vi "Simulated Thermocouple RT Driver VI.vi"(6 "Device Clock":string, 9 "Device Inputs FIFO":refnum<k33>, 10 "Device Outputs FIFO":refnum<k33>, 11 "Device Reference":T1 format="%.0x") -> ()   [LabVIEW 2011, in "Simulated Thermocouple Custom Device.lvlib"]
uses:
  Simulated Thermocouple Custom Device.lvlib
  <vilib>/NI Veristand/Custom Device API/Custom Device Item Ref.ctl
  <vilib>/NI Veristand/Custom Device API/Custom Device Channel Type.ctl
  RT TC Update State.ctl
  <vilib>/Platform/TimedLoop/XDataNode/timing_clust.ctl
  <vilib>/Platform/TimedLoop/XDataNode/nitl_modes.ctl
  <vilib>/Platform/TimedLoop/XDataNode/wakeup.ctl
  <vilib>/NI Veristand/Custom Device API/Message Response (String).ctl
  <vilib>/NI Veristand/Custom Device API/Message Response (Byte Array).ctl
  <vilib>/DAQmx/write.llb/DAQmx Write (Analog 1D DBL NChan 1Samp).vi
  <vilib>/DAQmx/miscellaneous.llb/DAQmx Fill In Error Info.vi
  <vilib>/Platform/TimedLoop/XDataNode/XDataNode.xnode
  <vilib>/NI Veristand/Custom Device API/Custom Device API.lvlib
  <vilib>/NI Veristand/Custom Device Tools/Custom Device Utility Library/Custom Device Utility Library.lvlib
  <vilib>/Platform/TimedLoop/XDataNode/XDNodeRunTimeDep.lvlib
panel:
  in  "Initialization Status Notifier":refnum<notifier>
  in  "Status Notifier":refnum<notifier>
  # "Custom Device Template\nv1.0"
  # "Use this template as a starting point for creating a custom device code module. The input controls shown here are specially named controls that the system will use to provide the device loop with data. The controls are not required for the device loop to run. For instance, if the device doesn't produce any output data, then you don't need the Device Outputs FIFO control. If you do use these controls, however, they need to have these exact names to be functional."
  # "The optional status notifier element is used to notify the RT engine of the last state of the custom device, and to indicate the device has completed execution. If this control is not used, a default No Error value is returned to the system when the device finishes execution.\n\nNote: This error state is not checked until the system shuts down. Use an output status channel to send more immediate status values to the system."
  # "This optional input can be used to send the VeriStand Engine the final status of the custom device initalization process. If this control exists on the custom device front panel, the VeriStand Engine will wait for a status update before starting up. If the custom device reports an error, that will abort the execution of the current configuration in the VeriStand Engine.\n\nThis control can be deleted if the custom device does not need to send the initialization status update."
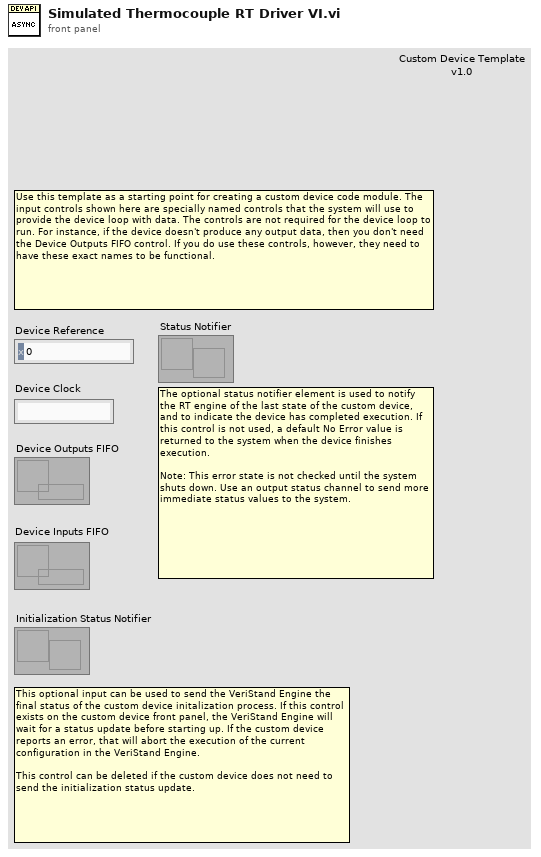
[diagram p1: front panel]
types:
  T1 = typedef "Custom Device API.lvlib/Custom Device Item Ref.ctl" = u64
  T2 = typedef "Custom Device API.lvlib/Custom Device Channel Type.ctl" = enum16{"Input", "Output"}
  T3 = typedef "Custom Device API.lvlib/Custom Device Timed Loop Priority.ctl" = enum32{"Low", "Medium", "High"}
  T4 = typedef "Custom Device API.lvlib/Custom Device Engine Event Ref.ctl" = refnum<event-registration>
  T5 = typedef "Simulated Thermocouple Custom Device.lvlib/RT Config Data.ctl" = cluster{"Current Task":refnum<k21>, "Voltage Task":refnum<k21>, "FIFO Sort Key":enum16{"SimTC", "Calibration", "VO", "CO"}[], "Cal Channel Indicies":i32[], "Current Initial Values":dbl[], "Voltage Initial Values":dbl[], "TC Channel Config":T6[], "TC Update Period":dbl, "Voltage Divider Ratio":dbl, "Samples To Collect":dbl, "Temperature Units":T8, "Cal Settling Time":dbl, "Cal Types":T7[]}
  T6 = typedef "Simulated Thermocouple Custom Device.lvlib/TC Channel Config Data.ctl" = cluster{"Thermocouple Type":T7, "Temperature Units":T8}
  T7 = typedef "Simulated Thermocouple Custom Device.lvlib/TC Selector.ctl" = u16
  T8 = typedef "Simulated Thermocouple Custom Device.lvlib/TC Unit Selector.ctl" = u16
  T9 = typedef "Simulated Thermocouple Custom Device.lvlib/RT TC Update State.ctl" = enum16{"Init", "Calibrate", "Update", "Idle"}
  T10 = typedef "XDNodeRunTimeDep.lvlib/timing_clust.ctl" = cluster{"Expected End [f-1]":u64, "Actual End [f-1]":u64, "Finished Late? [f-1]":bool, "Expected End [i-1]":u64, "Actual End [i-1]":u64, "Finished Late? [i-1]":bool, "Expected Start [i]":u64, "Actual Start [i]":u64, "Expected Start [f]":u64, "Actual Start [f]":u64, "Source Name":string, "Structure Name":string, "Period":i64, "Deadline":i64, "Offset":i64, "Start":i64, "Priority":i32, "Timeout":i32, "Mode":T11, "Wakeup Reason":T12, "Error":errorcluster, "Source Type":string, "Secondary Source Type":string, "Global End Time":u64, "Global Start Time":u64, "Frame Duration":u64, "Iteration Duration":u64, "Assigned CPU":i32, "I/O Scan Engine Mode":u32}
  T11 = typedef "XDNodeRunTimeDep.lvlib/nitl_modes.ctl" = enum32{"No Change", "Process missed periods, maintain original phase", "Discard missed periods, maintain original phase", "Process missed periods, ignore original phase", "Discard missed periods, ignore original phase"}
  T12 = typedef "XDNodeRunTimeDep.lvlib/wakeup.ctl" = enum32{"Normal", "Aborted", "Asynchronous wakeup", "Timing source error", "Timed loop error", "Timeout"}
  T13 = typedef "Custom Device API.lvlib/Message Response (String).ctl" = cluster{"Response":string, "Error":errorcluster}
  T14 = typedef "Custom Device API.lvlib/Message Response (Byte Array).ctl" = cluster{"Response":u8[], "Error":errorcluster}
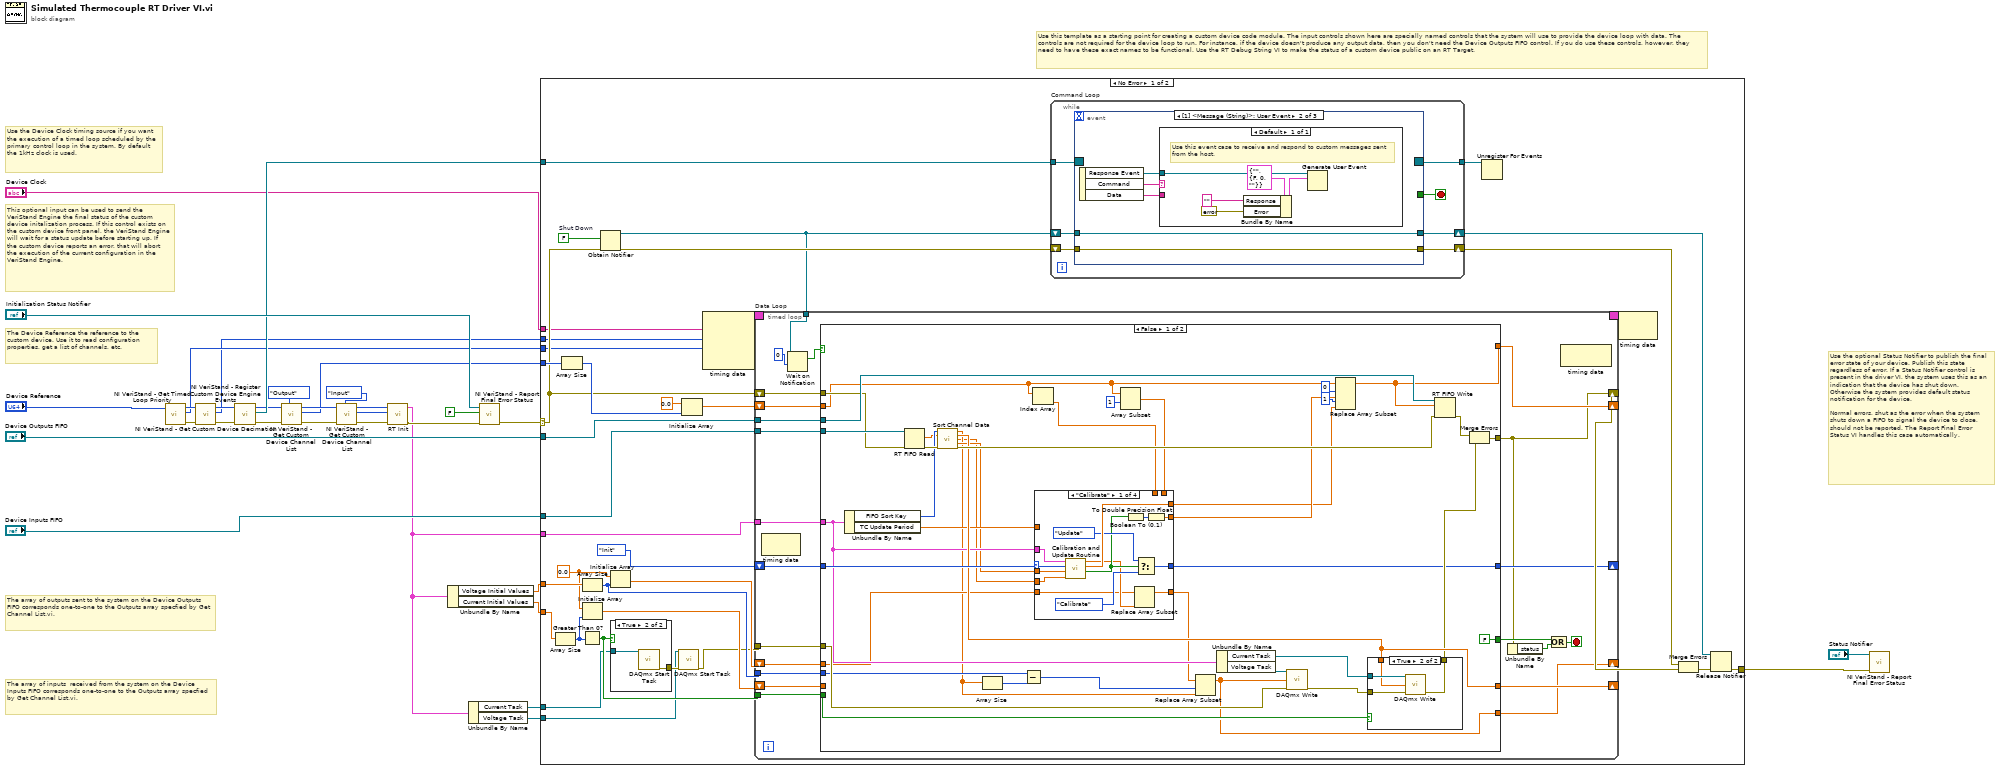
[diagram p0: block diagram]
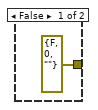
[diagram p2: hidden frame]
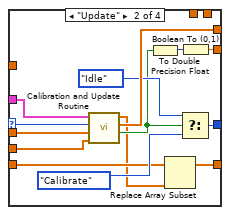
[diagram p4: hidden frame]
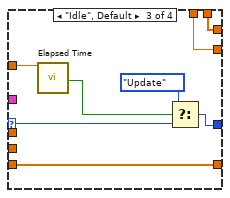
[diagram p5: hidden frame]
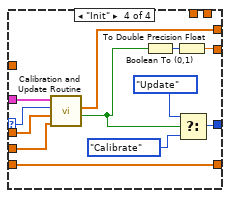
[diagram p6: hidden frame]
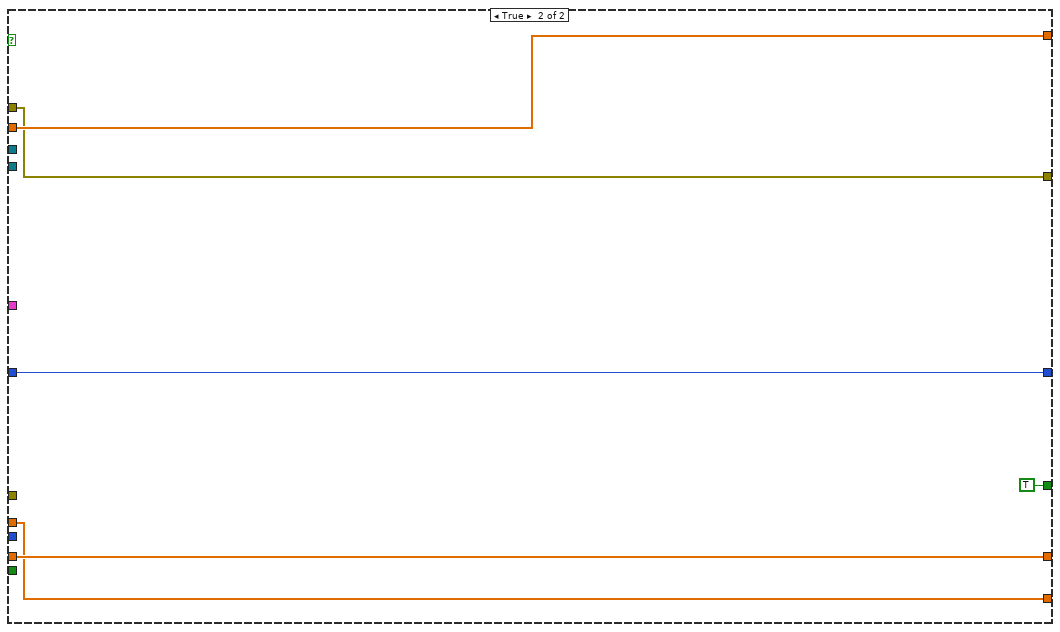
[diagram p7: hidden frame]
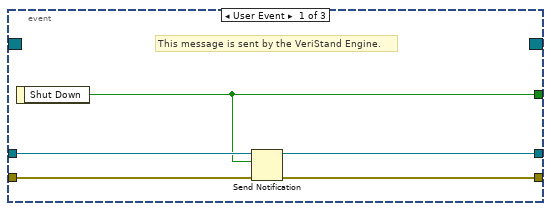
[diagram p8: hidden frame]
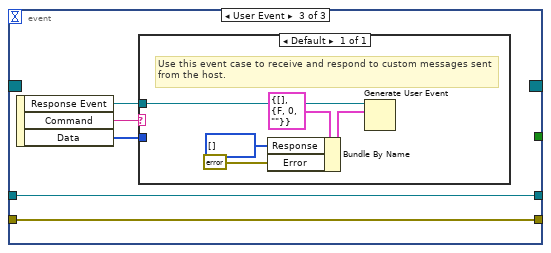
[diagram p9: hidden frame]
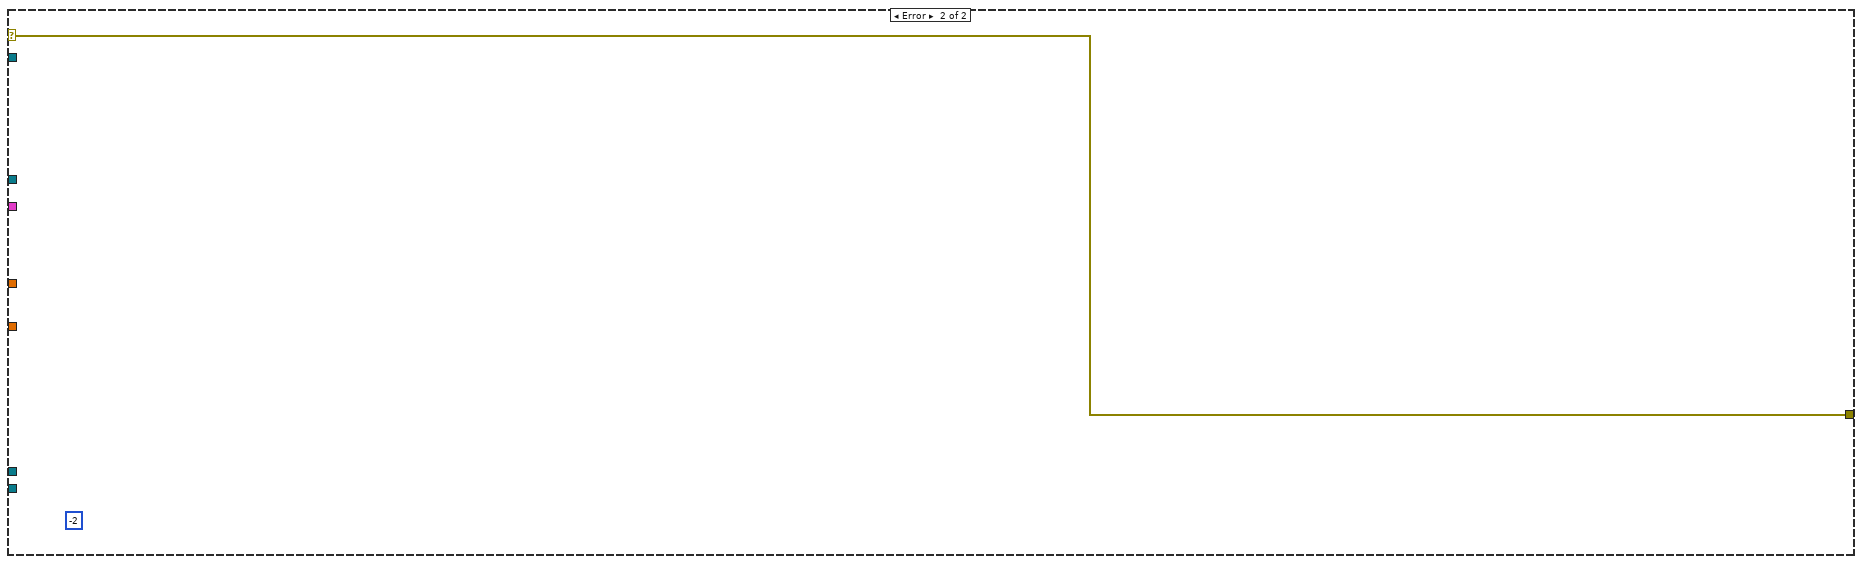
[diagram p10: hidden frame]
diagram:
  # "This optional input can be used to send the VeriStand Engine the final status of the custom device initalization process. If this control exists on the custom device front panel, the VeriStand Engine will wait for a status update before starting up. If the custom device reports an error, that will abort the execution of the current configuration in the VeriStand Engine."
  # "The array of inputs  received from the system on the Device Inputs FIFO corresponds one-to-one to the Outputs array specfied by Get Channel List.vi."
  # "Use the optional Status Notifier to publish the final error state of your device. Publish this state regardless of error. If a Status Notifier control is present in the driver VI, the system uses this as an indication that the device has shut down. Otherwise the system provides default status notification for the device.\n\nNormal errors, shut as the error when the system shuts down a FIFO to signal the device to close, should not be reported. The Report Final Error Status VI handles this case automatically."
  # "The array of outputs sent to the system on the Device Outputs FIFO corresponds one-to-one to the Outputs array specfied by Get Channel List.vi."
  # "The Device Reference the reference to the custom device. Use it to read configuration properties, get a list of channels, etc."
  # "Use the Device Clock timing source if you want the execution of a timed loop scheduled by the primary control loop in the system. By default the 1kHz clock is used."
  # "Use this template as a starting point for creating a custom device code module. The input controls shown here are specially named controls that the system will use to provide the device loop with data. The controls are not required for the device loop to run. For instance, if the device doesn't produce any output data, then you don't need the Device Outputs FIFO control. If you do use these controls, however, they need to have these exact names to be functional. Use the RT Debug String VI to make the status of a custom device public on an RT Target."
  n1 = call <vilib>:"NI VeriStand - Get Timed Loop Priority.vi"("Device Ref in"="Device Reference") -> ("error out"=w16:errorcluster, "Priority"=w4:T3, "Device Ref out"=w15:T1)  [unwired: 8 in]
  n2 = call <vilib>:"NI VeriStand - Get Custom Device Decimation.vi"("error in (no error)"=w16, "Device Ref in"=w15) -> ("error out"=w18:errorcluster, "Decimation"=w3:i32, "Device Ref out"=w17:T1)  [unwired: 7 in]
  n3 = call <vilib>:"NI VeriStand - Register Custom Device Engine Events.vi"("error in (no error)"=w18, "Device Ref in"=w17) -> ("error out"=w32:errorcluster, "Custom Device Engine Event Ref"=w23:T4, "Device Ref out"=w21:T1)  [unwired: 7 in]
  n4 = call <vilib>:"NI VeriStand - Get Custom Device Channel List.vi"("Channel Type"=Custom_Device_Channel_Type."Output", "error in (no error)"=w32, "Device Ref in"=w21) -> ("error out"=w26:errorcluster, "Specified Channel Ref List"=w19:T1[], "Device Ref out"=w27:T1)  [unwired: 6 out]
  n5 = call <vilib>:"NI VeriStand - Get Custom Device Channel List.vi"("Channel Type"=Custom_Device_Channel_Type."Input", "error in (no error)"=w26, "Device Ref in"=w27) -> ("error out"=w14:errorcluster, "Specified Channel Ref List"=w11:T1[], "Device Ref out"=w12:T1)  [unwired: 6 out]
  n6 = call "RT Init.vi"("error in"=w14, "Input Channels"=w11, "Custom Device Ref in"=w12) -> ("error out"=w13:errorcluster, "RT Configuration Data"=w7:T5)  [unwired: 7 in]
  n7 = Unbundle By Name(w7) -> ("Voltage Initial Values"=w9:dbl[], "Current Initial Values"=w8:dbl[])
  n8 = Unbundle By Name(w7) -> ("Current Task"=w6:refnum<k21>, "Voltage Task"=w5:refnum<k21>)
  n9 = call <vilib>:"NI VeriStand - Report Final Error Status.vi"("error in (no error)"=w13, "Filter FIFO Errors (T)"=FALSE, "Status Notifier"="Initialization Status Notifier") -> ("error out"=w20:errorcluster)  [unwired: 8 out]
  n10 = case shown="No Error" w20 {
    selector: w20 -> [w43 w232]
    tunnel: "Device Outputs FIFO" -> [w67 _]
    tunnel: "Device Inputs FIFO" -> [w66 _]
    tunnel: w19 -> [w62 _]
    tunnel: w23 -> [w61 _]
    tunnel: [w59 w232] -> w22
    tunnel: w7 -> [w41 _]
    tunnel: w9 -> [w50 _]
    tunnel: w8 -> [w49 _]
    tunnel: w6 -> [w37 _]
    tunnel: w5 -> [w36 _]
    tunnel: "Device Clock" -> [w35 _]
    tunnel: w4 -> [w34 _]
    tunnel: w3 -> [w33 _]
    frame No Error {
      w48 = 0.0 ("element")
      w60 = FALSE  # Shut Down
      n11 = Array Size(array=w49) -> (size(s)=w45:i32)
      n12 = Array Size(array=w62) -> (size(s)=w63:i32)
      n13 = Greater Than 0?(x=w45) -> (x > 0?=w38:bool)
      n14 = Array Size(array=w50) -> (size(s)=w44:i32)
      n15 = Initialize Array(w48, w45) -> (w46:dbl[])
      n16 = Obtain Notifier(notification data type=w60, error in (no error)=w43) -> (notifier out=w57:refnum<notifier>, error out=w68:errorcluster)  [unwired: 2 in, 1 out]
      n17 = Initialize Array(w48, w44) -> (w47:dbl[])
      n18 = case shown="True" w38 {
        tunnel: [errorcluster {"status"=FALSE, "code"=0, "source"=""} ("error out") w71] -> w39
        tunnel: w37 -> [_ w70]
        frame False {
        }
        frame True {
          n19 = call <vilib>:"DAQmx Start Task.vi"("task/channels in"=w70) -> ("error out"=w71:errorcluster)  [unwired: 13 in, 1 out]
        }
      }
      n20 = call <vilib>:"DAQmx Start Task.vi"("task/channels in"=w36, "error in"=w39) -> ("error out"=w40:errorcluster)  [unwired: 12 in, 1 out]
      n21 = Initialize Array(0.0 ("element"), w63) -> (w64:dbl[])
      n22 = node-c288(w35, w33, w34) -> (w53:T10)  [unwired: 1 in]
      n23 = timed-loop "Data Loop" {
        shift-right: [w92] -> _
        shift-left: w64 -> [w93]
        tunnel: w67 -> [w91]
        tunnel: w66 -> [w90]
        tunnel: w57 -> [w88]
        timing: w53 -> [_]
        timing-out: [_] -> w52
        tunnel: w41 -> [w85]
        shift-right: [w78] -> _
        shift-left: RT_TC_Update_State."Init" ("Enum") -> [w83]
        shift-right: [w79] -> _
        shift-left: w47 -> [w82]
        shift-right: [w80] -> _
        shift-left: w46 -> [w76]
        tunnel: w38 -> [w84]
        tunnel: w44 -> [w81]
        shift-right: [w75] -> w42
        shift-left: w43 -> [w77]
        tunnel: w40 -> [w73]
        stop <- w74 stop-if-true
        n24 = node-c288() -> ()  [unwired: 1 in, 1 out]
        n25 = Wait on Notification(notifier=w88, timeout in ms (-1)=0) -> (notification=w87:bool)  [unwired: 2 in, 3 out]
        n26 = case shown="False" w87 {
          tunnel: w93 -> [w110 w193]
          tunnel: [w114 w193] -> w92
          tunnel: w91 -> [w134 _]
          tunnel: w90 -> [w133 _]
          tunnel: [FALSE TRUE] -> w86
          tunnel: w85 -> [w117 _]
          tunnel: [w121 w191] -> w75
          tunnel: w84 -> [w128 _]
          tunnel: w83 -> [w126 w190]
          tunnel: w82 -> [w111 w188]
          tunnel: w81 -> [w100 _]
          tunnel: [w125 w189] -> w80
          tunnel: [w101 w188] -> w79
          tunnel: [w105 w190] -> w78
          tunnel: w77 -> [w122 w191]
          tunnel: w76 -> [_ w189]
          tunnel: w73 -> [w118 _]
          frame False {
            n27 = Unbundle By Name(w117) -> ("FIFO Sort Key"=w130:enum16{"SimTC", "Calibration", "VO", "CO"}[], "TC Update Period"=w123:dbl)
            n28 = RT FIFO Read(0:w133, 3:w122) -> (9:w113:dbl[], 11:w132:errorcluster)  [unwired: 1 in, 4 out]
            n29 = call "Sort Channel Data.vi"("Key"=w130, "Input Data"=w113, "error in (no error)"=w132) -> ("VO Channels"=w99:dbl[], "CO Channels"=w125:dbl[], "SimTC Channels"=w96:dbl[], "Calibration Channels"=w103:dbl[], "error out"=w129:errorcluster)  [unwired: 8 in]
            n30 = Array Size(array=w99) -> (size(s)=w98:i32)
            n31 = Subtract(x=w100, y=w98) -> (x-y=w97:i32)
            n32 = Index Array(array=w110) -> (element=w107:dbl)  [unwired: 1 in]
            n33 = Array Subset(array=w110, index=1) -> (w108:dbl[])  [unwired: 1 in]
            n34 = case shown="\"Calibrate\"" w126 {
              selector: w126 -> [w153 w166 w174 w186]
              tunnel: w111 -> [w140 w155 w168 w183]
              tunnel: [w142 w156 w168 w183] -> w102
              tunnel: w123 -> [_ _ w175 _]
              tunnel: [w147 w158 w171 w176] -> w105
              tunnel: w96 -> [w150 w164 _ w184]
              tunnel: w117 -> [w152 w167 _ w187]
              tunnel: w103 -> [w151 w165 _ w185]
              tunnel: [w149 w163 w169 w182] -> w104
              tunnel: [w143 w162 w170 w180] -> w106
              tunnel: w108 -> [_ _ w169 _]
              tunnel: w107 -> [_ _ w170 _]
              frame "Calibrate" {
                n35 = call "Calibration and Update Routine.vi"("simTC Channels"=w150, "Cal Channels"=w151, "TC Update State"=w153, "RT Configuration Data"=w152) -> ("Cal Valid?"=w145:bool, "Error"=w149:dbl[], "Voltages to Output"=w141:dbl[])  [unwired: 5 in]
                n36 = Boolean To (0,1)(Boolean=w145) -> (0, 1=w144:i16)
                n37 = Replace Array Subset(array=w140, new element=w141) -> (w142:dbl[])  [unwired: 1 in]
                n38 = Select(t=RT_TC_Update_State."Update" ("Enum"), s=w145, f=RT_TC_Update_State."Calibrate") -> (s? t:f=w147:T9)
                n39 = To Double Precision Float(number=w144) -> (double precision float=w143:dbl)
              }
              frame "Update" {
                n40 = call "Calibration and Update Routine.vi"("simTC Channels"=w164, "Cal Channels"=w165, "TC Update State"=w166, "RT Configuration Data"=w167) -> ("Cal Valid?"=w159:bool, "Error"=w163:dbl[], "Voltages to Output"=w154:dbl[])  [unwired: 5 in]
                n41 = Boolean To (0,1)(Boolean=w159) -> (0, 1=w161:i16)
                n42 = Replace Array Subset(array=w155, new element=w154) -> (w156:dbl[])  [unwired: 1 in]
                n43 = Select(t=RT_TC_Update_State."Idle" ("Enum"), s=w159, f=RT_TC_Update_State."Calibrate") -> (s? t:f=w158:T9)
                n44 = To Double Precision Float(number=w161) -> (double precision float=w162:dbl)
              }
              frame "Idle", Default {
                n45 = call "Elapsed Time"("Time Target (s)"=w175) -> ("Time has Elapsed"=w172:bool)  [unwired: 11 in, 7 out]
                n46 = Select(t=RT_TC_Update_State."Update", s=w172, f=w174) -> (s? t:f=w171:T9)
              }
              frame "Init" {
                n47 = call "Calibration and Update Routine.vi"("simTC Channels"=w184, "Cal Channels"=w185, "TC Update State"=w186, "RT Configuration Data"=w187) -> ("Cal Valid?"=w177:bool, "Error"=w182:dbl[])  [unwired: 5 in, 1 out]
                n48 = Boolean To (0,1)(Boolean=w177) -> (0, 1=w181:i16)
                n49 = To Double Precision Float(number=w181) -> (double precision float=w180:dbl)
                n50 = Select(t=RT_TC_Update_State."Update", s=w177, f=RT_TC_Update_State."Calibrate" ("Enum")) -> (s? t:f=w176:T9)
              }
            }
            n51 = Replace Array Subset(array=w102, new element=w99, index=w97) -> (w101:dbl[])
            n52 = Unbundle By Name(w117) -> ("Current Task"=w127:refnum<k21>, "Voltage Task"=w124:refnum<k21>)
            n53 = call-poly <vilib>:"DAQmx Write.vi"("task/channels in"=w124, "data"=w101, "error in"=w118) -> ("error out"=w112:errorcluster)  [unwired: 10 in, 2 out]
            n54 = Replace Array Subset(array=w110, new element #1=w106, index #1=0 ("index"), new element #2=w104, index #2=1 ("index")) -> (w114:dbl[])
            n55 = case shown="True" w128 {
              tunnel: w127 -> [_ w139]
              tunnel: w125 -> [_ w138]
              tunnel: w112 -> [w135 w137]
              tunnel: [w135 w136] -> w119
              frame False {
              }
              frame True {
                n56 = call-poly <vilib>:"DAQmx Write.vi"("task/channels in"=w139, "data"=w138, "error in"=w137) -> ("error out"=w136:errorcluster)  [unwired: 10 in, 2 out]
              }
            }
            n57 = RT FIFO Write(0:w134, 1:w114, 3:w129) -> (11:w120:errorcluster)  [unwired: 1 in, 4 out]
            n58 = Merge Errors(w120, w119) -> (w121:errorcluster)
          }
          frame True {
          }
        }
        n59 = Unbundle By Name(w75) -> ("status"=w72:bool)
        n60 = Compound Arithmetic op=OR(w86, w72) -> (w74:bool)
        n61 = node-c288() -> ()  [unwired: 1 in, 1 out]
      }
      n62 = while "Command Loop" {
        tunnel: w61 -> [w206]
        tunnel: [w205] -> w58
        shift-right: [w202] -> w56
        shift-left: w57 -> [w203]
        shift-right: [w200] -> w54
        shift-left: w68 -> [w201]
        stop <- w204 stop-if-true
        n63 = event shown="[1] <Message (String)>: User Event" {
          selector: w206 -> [_ _ _]
          dyn-events: [_ _ _] -> w205
          timeout: _ -> [_ _ _]
          tunnel: [w209 _ _] -> w204
          tunnel: w203 -> [w210 w214 w224]
          tunnel: [w211 w214 w224] -> w202
          tunnel: w201 -> [w208 w212 w222]
          tunnel: [w207 w212 w222] -> w200
          event User Event {
            # "This message is sent by the VeriStand Engine."
            n64 = event-data() -> ("Shut Down"=w209:bool)  [unwired: 1 in]
            n65 = Send Notification(notification=w209, notifier=w210, error in (no error)=w208) -> (notifier out=w211:refnum<notifier>, error out=w207:errorcluster)
          }
          event User Event {
            n66 = event-data() -> ("Response Event"=w213:refnum<user-event>, "Command"=w216:string, "Data"=w215:string)  [unwired: 1 in]
            n67 = case shown="Default" w216 {
              tunnel: w215 -> [_]
              tunnel: w213 -> [w221]
              frame Default {
                # "Use this event case to receive and respond to custom messages sent from the host."
                n68 = Bundle By Name(cluster=T13 {"Response"="", "Error"={"status"=FALSE, "code"=0, "source"=""}} ("event data"), "Response"="", "Error"=errorcluster {"status"=FALSE, "code"=0, "source"=""}) -> (w219:T13)
                n69 = Generate User Event(user event=w221, event data cluster=w219) -> ()  [unwired: 1 in, 2 out]
              }
            }
          }
          event User Event {
            n70 = event-data() -> ("Response Event"=w223:refnum<user-event>, "Command"=w226:string, "Data"=w225:u8[])  [unwired: 1 in]
            n71 = case shown="Default" w226 {
              tunnel: w225 -> [_]
              tunnel: w223 -> [w231]
              frame Default {
                # "Use this event case to receive and respond to custom messages sent from the host."
                n72 = Bundle By Name(cluster=T14 {"Response"=[], "Error"={"status"=FALSE, "code"=0, "source"=""}} ("event data"), "Response"=u8[] [], "Error"=errorcluster {"status"=FALSE, "code"=0, "source"=""}) -> (w228:T14)
                n73 = Generate User Event(user event=w231, event data cluster=w228) -> ()  [unwired: 1 in, 2 out]
              }
            }
          }
        }
      }
      n74 = Unregister For Events(event registration refnum=w58) -> ()  [unwired: 1 in, 1 out]
      n75 = node-c288(w52) -> ()  [unwired: 1 out]
      n76 = Merge Errors(w54, w42) -> (w55:errorcluster)
      n77 = Release Notifier(notifier=w56, error in (no error)=w55) -> (error out=w59:errorcluster)  [unwired: 1 in, 2 out]
    }
    frame Error {
      (unwired) -2
    }
  }
  n78 = call <vilib>:"NI VeriStand - Report Final Error Status.vi"("error in (no error)"=w22, "Status Notifier"="Status Notifier") -> ()  [unwired: 1 in, 9 out]
